vi "Logger Check and Write.vi"(8 "error in (no error)":errorcluster, 11 "RDS Logger Actor in":refnum<class "RDS Logger Actor.lvclass">) -> (0 "error out":errorcluster, 3 "RDS Logger Actor out":refnum<class "RDS Logger Actor.lvclass">)   [LabVIEW 2015, in "RDS Logger Actor.lvlib" / "RDS Logger Actor.lvclass"]
uses:
  RDS Logger Actor.lvclass
  RDS Logger Actor.lvclass/RDS Logger Actor.ctl
  RDS State Tracker/RDS State/RDS State.lvclass
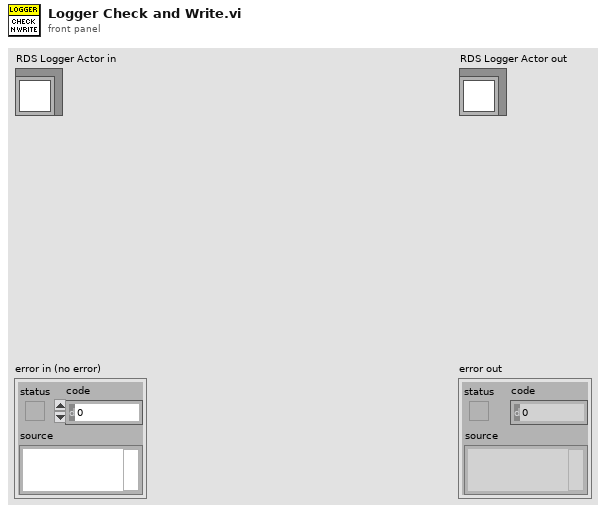
[diagram p1: front panel]
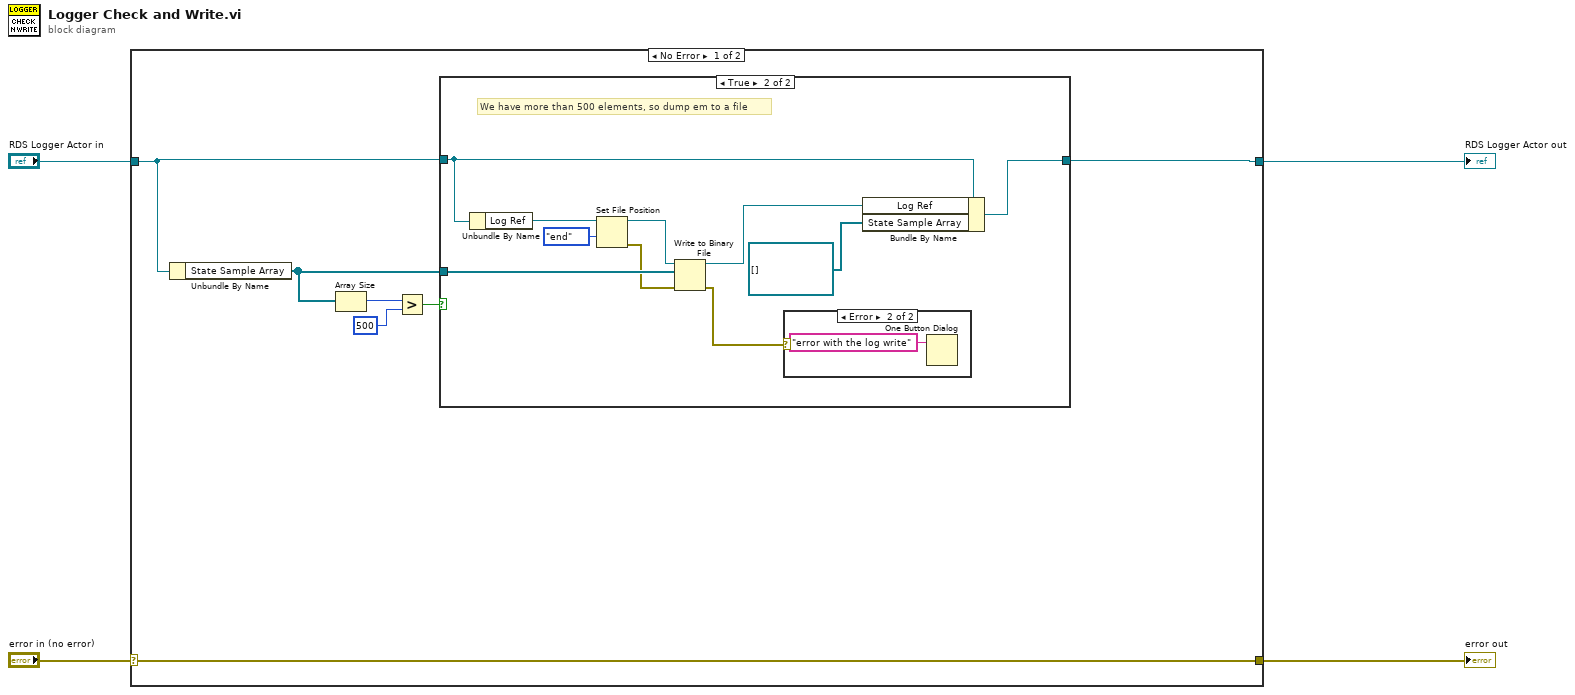
[diagram p0: block diagram]
diagram:
  n1 = case shown="No Error" "error in (no error)" {
    selector: "error in (no error)" -> [w11 w25]
    tunnel: [w11 w25] -> w3
    tunnel: [w6 w24] -> w1
    tunnel: "RDS Logger Actor in" -> [w7 w24]
    frame No Error {
      n2 = Unbundle By Name(w7) -> ("State Sample Array"=w8:refnum<class "RDS State.lvclass">[])
      n3 = Array Size(array=w8) -> (size(s)=w10:i32)
      n4 = Greater?(x=w10, y=500) -> (0:w5:bool)
      n5 = case shown="True" w5 {
        tunnel: w8 -> [_ w22]
        tunnel: w7 -> [w12 w17]
        tunnel: [w12 w15] -> w6
        frame False {
        }
        frame True {
          # "We have more than 500 elements, so dump em to a file"
          n6 = Unbundle By Name(w17) -> ("Log Ref"=w21:refnum<file>)
          n7 = Set File Position(refnum=w21, from (0:start)=enum16{"start", "end", "current"}."end") -> (refnum out=w19:refnum<file>, error out=w18:errorcluster)  [unwired: 2 in]
          n8 = Write to Binary File(file (use dialog)=w19, data=w22, error in=w18) -> (refnum out=w13:refnum<file>, error out=w14:errorcluster)  [unwired: 3 in, 1 out]
          n9 = case shown="Error" w14 {
            frame No Error {
            }
            frame Error {
              n10 = One Button Dialog(message="error with the log write") -> ()  [unwired: 1 in, 1 out]
            }
          }
          n11 = Bundle By Name(cluster=w17, "Log Ref"=w13, "State Sample Array"=refnum<class "RDS State.lvclass">[] []) -> (w15:refnum<class "RDS Logger Actor.lvclass">)
        }
      }
    }
    frame Error {
    }
  }
  "error out" <- w3
  "RDS Logger Actor out" <- w1
